vi "reInitCount.vi"(8 "Error In":errorcluster, 11 "Production Date":string) -> (0 "Error Out":errorcluster, 3 "Count":string)   [LabVIEW 2018]
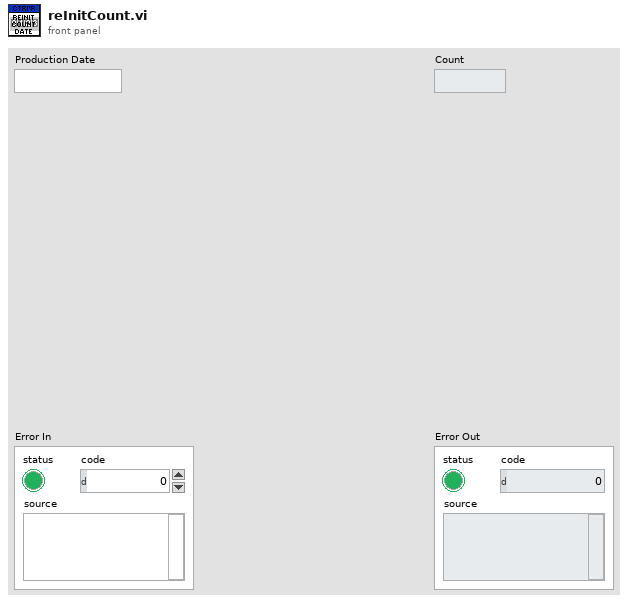
[diagram p1: front panel]
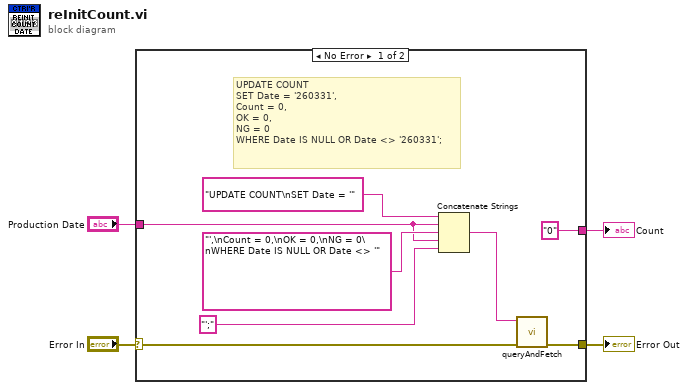
[diagram p0: block diagram]
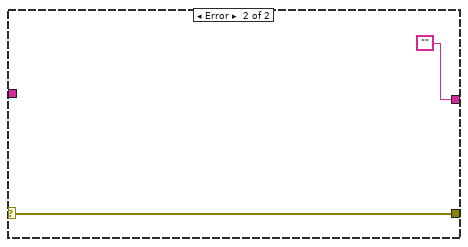
[diagram p2: hidden frame]
diagram:
  n1 = case shown="No Error" "Error In" {
    selector: "Error In" -> [w12 w14]
    tunnel: [w11 w14] -> w3
    tunnel: "Production Date" -> [w8 _]
    tunnel: ["0" ""] -> w1
    frame No Error {
      # "UPDATE COUNT\nSET Date = '260331',\nCount = 0,\nOK = 0,\nNG = 0\nWHERE Date IS NULL OR Date <> '260331';"
      n2 = Concatenate Strings("UPDATE COUNT\nSET Date = '", w8, "',\nCount = 0,\nOK = 0,\nNG = 0\nWHERE Date IS NULL OR Date <> '", w8, "';") -> (w6:string)
      n3 = call "queryAndFetch.vi"("Error In"=w12, "Query"=w6) -> ("Error Out"=w11:errorcluster)  [unwired: 8 in, 1 out]
    }
    frame Error {
    }
  }
  "Error Out" <- w3
  "Count" <- w1
